vi "GetRegisterOffset.vi"(8 "error in (no error)":errorcluster, 11 "element in":T1 {"Data Type" format="%.0x"}) -> (0 "error out":errorcluster, 2 "status":i32, 3 "element out":T1 {"Data Type" format="%.0x"})   [LabVIEW 2020, in "FPGA Addon Engine.lvlib"]
uses:
  FPGA Addon Engine.lvlib
  Types/Register Settings.ctl
  Addon Shared/Types/FPGA Addon Data Type.ctl
  Addon Shared/Types/Scalar Type.ctl
  NiFpga.dll
  Addon Shared/FPGA Addon Shared.lvlib
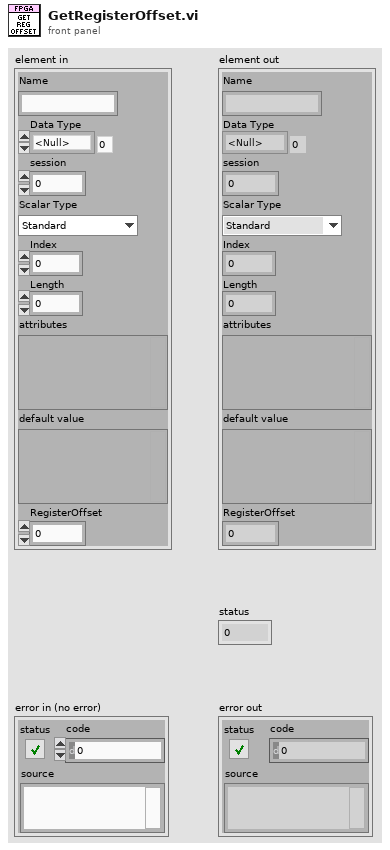
[diagram p1: front panel]
types:
  T1 = typedef "FPGA Addon Engine.lvlib/Register Settings.ctl" = cluster{"Name":string, "Data Type":T2, "session":u32, "Scalar Type":T3, "Index":i32, "Length":i32, "attributes":variant, "default value":variant, "RegisterOffset":u32}
  T2 = typedef "FPGA Addon Shared.lvlib/FPGA Addon Data Type.ctl" = enum8{"<Null>", "I8", "I16", "I32", "I64", "U8", "U16", "U32", "U64", "SGL", "Boolean", "Analog PWM In Settings", "Analog PWM In", "Digital PWM In Settings", "Digital PWM In", "Digital PWM Out", "Sine Out", "FXP", "FXP+/-24.5", "FXP+/-16.5", "FXP+/-32.8", "FXP+/-64.32", "FXP+/-16.7", "FXP+/-20.5", "FXP+/-27.5", "FXP+/-32.16", "FXP+16.3", "FXP+18.3", "Digital Static In", "Digital Static Out", "Digital Static In Settings", "Digital WSS Out", "Quad Encoder Settings", "Quad Encoder In", "Group"}
  T3 = typedef "FPGA Addon Shared.lvlib/Scalar Type.ctl" = enum16{"Standard", "Bitpacked"}
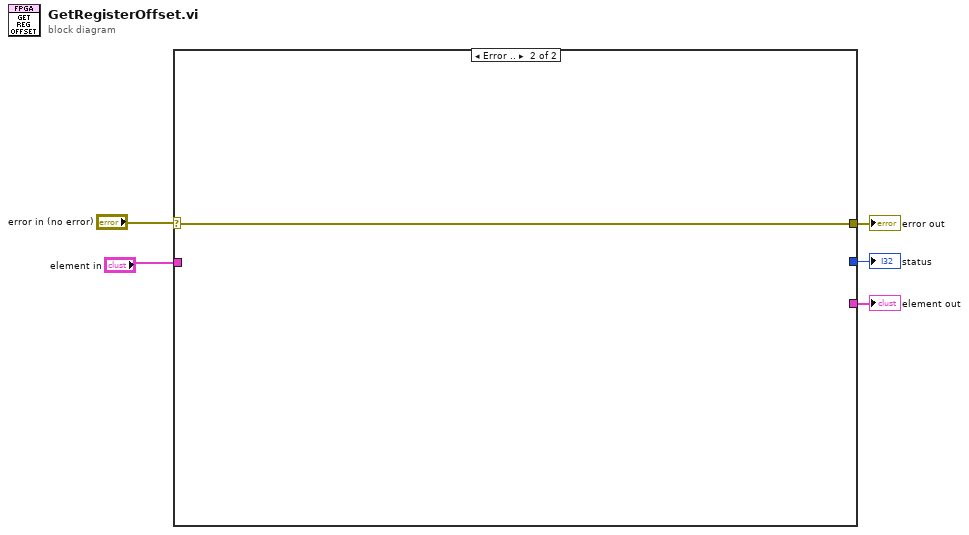
[diagram p0: block diagram]
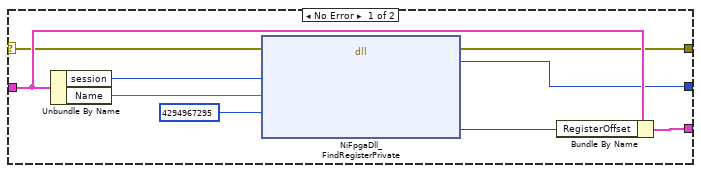
[diagram p2: hidden frame]
diagram:
  n1 = case shown="Error .." "error in (no error)" {
    selector: "error in (no error)" -> [w6 w15]
    tunnel: "element in" -> [w12 _]
    tunnel: [w10 w15] -> w4
    tunnel: [w8 _] -> w2
    tunnel: [w7 _] -> w1
    frame No Error {
      n2 = Unbundle By Name(w12) -> ("session"=w14:u32, "Name"=w13:string)
      n3 = dll-call lib="NiFpga.*" fn="NiFpgaDll_FindRegisterPrivate"(error in=w6, "session"=w14, "registerName"=w13, "expectedResourceType"=u32 4294967295) -> (error out=w10:errorcluster, "status"=w7:i32, "resourceOffset"=w11:u32)  [unwired: 6 in, 1 out]
      n4 = Bundle By Name(cluster=w12, "RegisterOffset"=w11) -> (w8:T1)
    }
    frame Error {
    }
  }
  "error out" <- w4
  "element out" <- w2
  "status" <- w1
